vi "NumberDetector.vi"(1 "Array":dbl[](array[numeric])) -> (0 "f":string)   [LabVIEW 2020]
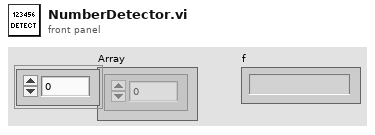
[diagram p1: front panel]
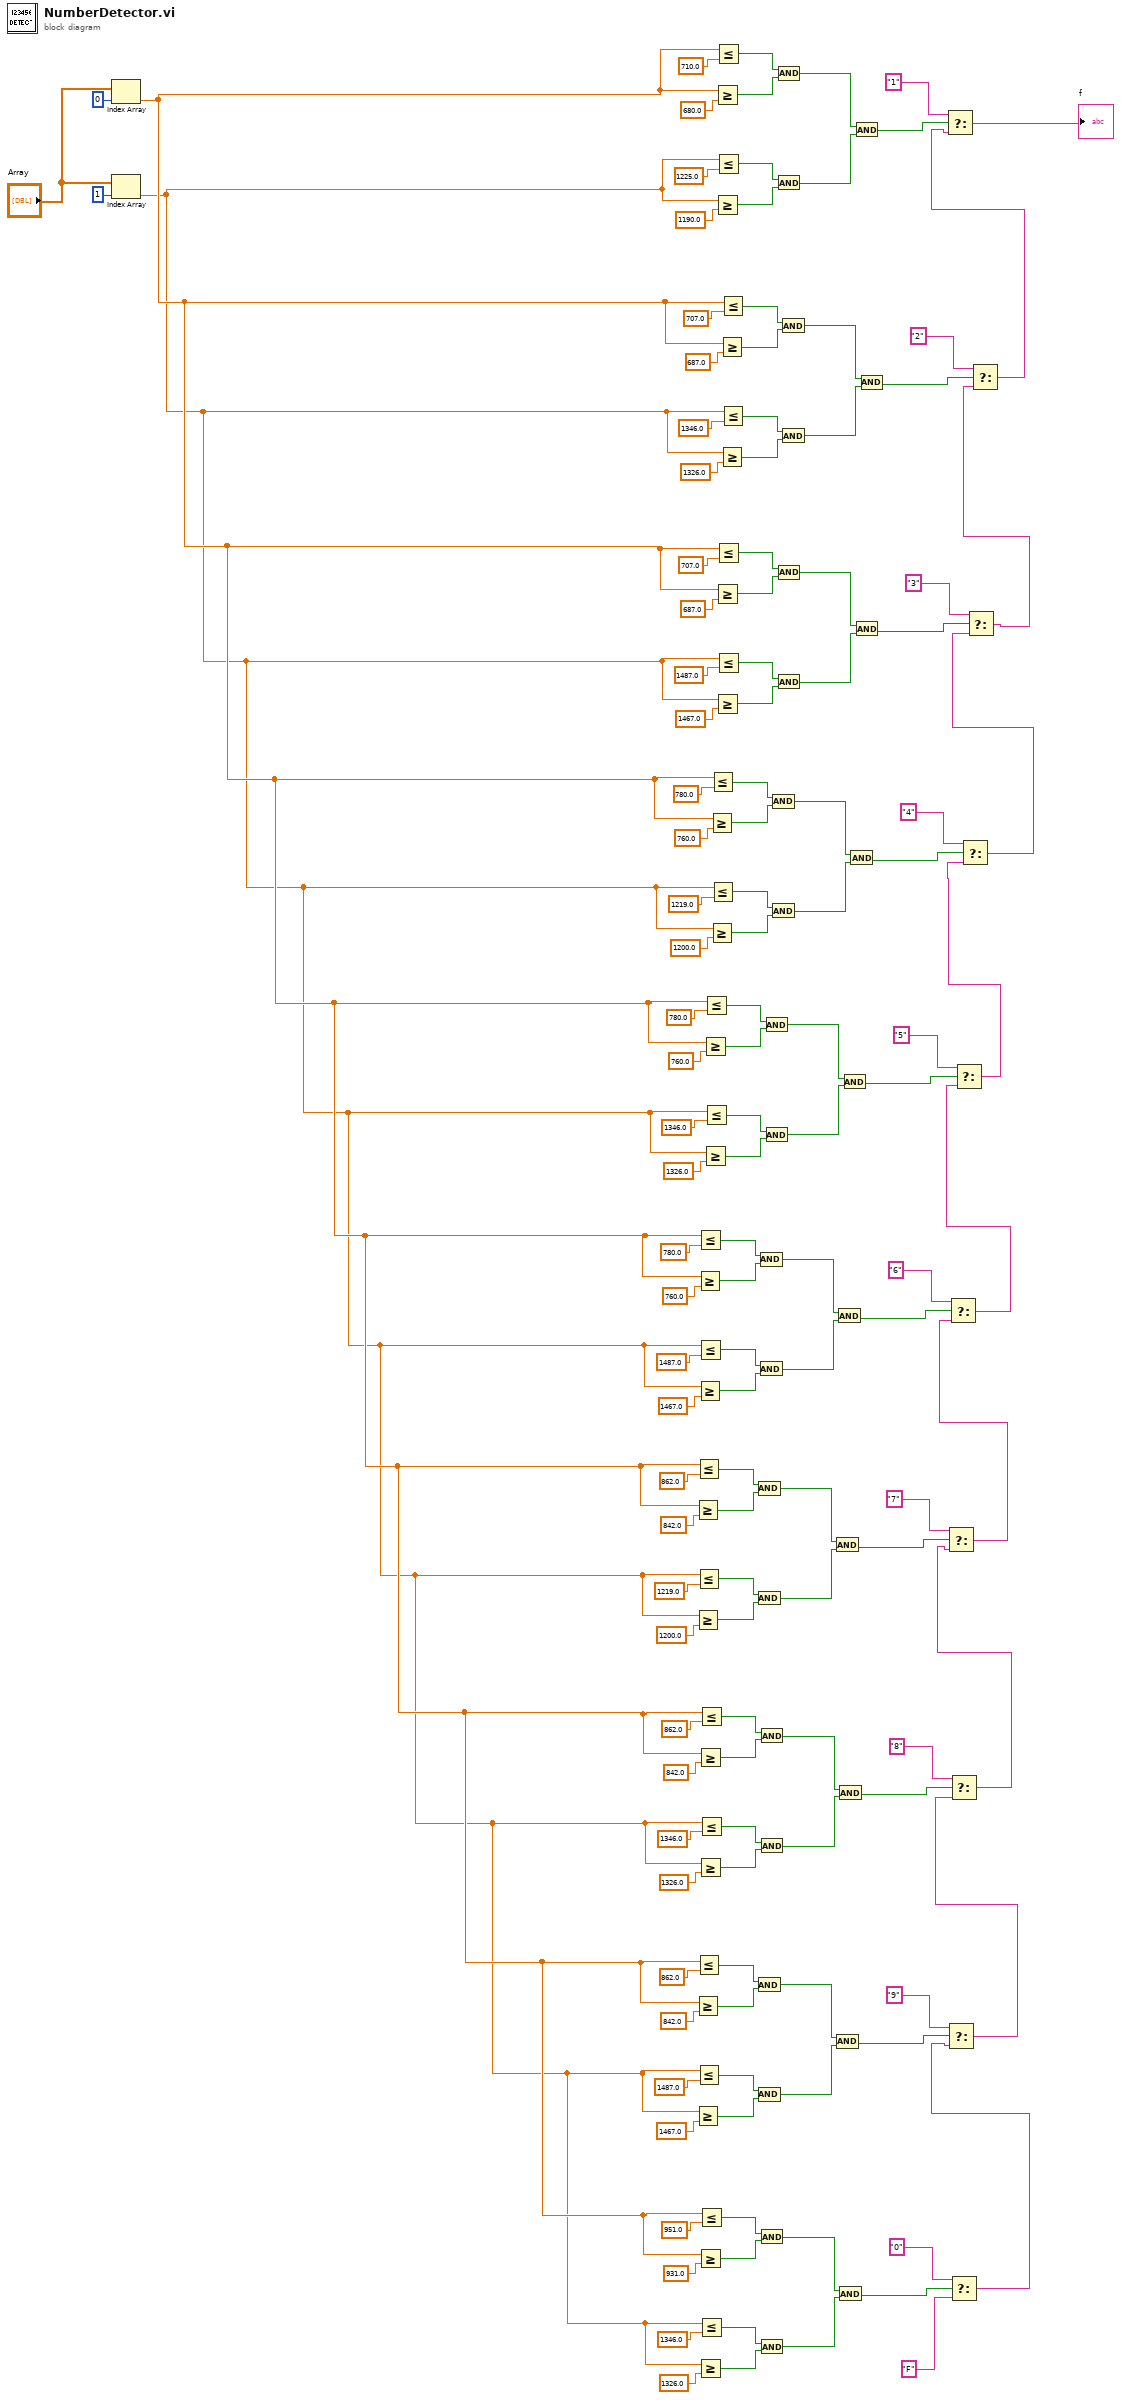
[diagram p0: block diagram]
diagram:
  n1 = Index Array(array="Array", index=0) -> (element=w4:dbl)
  n2 = Index Array(array="Array", index=1) -> (element=w3:dbl)
  n3 = Greater Or Equal?(x=w4, y=842.0) -> (x >= y?=w49:bool)
  n4 = Greater Or Equal?(x=w3, y=1200.0) -> (x >= y?=w50:bool)
  n5 = Greater Or Equal?(x=w4, y=842.0) -> (x >= y?=w23:bool)
  n6 = Greater Or Equal?(x=w3, y=1467.0) -> (x >= y?=w24:bool)
  n7 = Less Or Equal?(x=w4, y=862.0) -> (x <= y?=w48:bool)
  n8 = Less Or Equal?(x=w3, y=1219.0) -> (x <= y?=w51:bool)
  n9 = Less Or Equal?(x=w4, y=862.0) -> (x <= y?=w22:bool)
  n10 = Less Or Equal?(x=w3, y=1487.0) -> (x <= y?=w25:bool)
  n11 = Greater Or Equal?(x=w4, y=760.0) -> (x >= y?=w63:bool)
  n12 = Greater Or Equal?(x=w3, y=1467.0) -> (x >= y?=w62:bool)
  n13 = Less Or Equal?(x=w4, y=780.0) -> (x <= y?=w64:bool)
  n14 = Less Or Equal?(x=w3, y=1487.0) -> (x <= y?=w61:bool)
  n15 = Greater Or Equal?(x=w4, y=842.0) -> (x >= y?=w37:bool)
  n16 = Greater Or Equal?(x=w3, y=1326.0) -> (x >= y?=w36:bool)
  n17 = Greater Or Equal?(x=w4, y=931.0) -> (x >= y?=w11:bool)
  n18 = Greater Or Equal?(x=w3, y=1326.0) -> (x >= y?=w10:bool)
  n19 = Less Or Equal?(x=w4, y=862.0) -> (x <= y?=w38:bool)
  n20 = Less Or Equal?(x=w3, y=1346.0) -> (x <= y?=w35:bool)
  n21 = Less Or Equal?(x=w4, y=951.0) -> (x <= y?=w12:bool)
  n22 = Less Or Equal?(x=w3, y=1346.0) -> (x <= y?=w9:bool)
  n23 = Greater Or Equal?(x=w4, y=760.0) -> (x >= y?=w75:bool)
  n24 = Greater Or Equal?(x=w3, y=1326.0) -> (x >= y?=w76:bool)
  n25 = Less Or Equal?(x=w4, y=780.0) -> (x <= y?=w74:bool)
  n26 = Less Or Equal?(x=w3, y=1346.0) -> (x <= y?=w77:bool)
  n27 = Greater Or Equal?(x=w4, y=760.0) -> (x >= y?=w89:bool)
  n28 = Greater Or Equal?(x=w3, y=1200.0) -> (x >= y?=w88:bool)
  n29 = Less Or Equal?(x=w4, y=780.0) -> (x <= y?=w90:bool)
  n30 = Less Or Equal?(x=w3, y=1219.0) -> (x <= y?=w87:bool)
  n31 = Greater Or Equal?(x=w4, y=680.0) -> (x >= y?=w114:bool)
  n32 = Greater Or Equal?(x=w3, y=1190.0) -> (x >= y?=w115:bool)
  n33 = Greater Or Equal?(x=w4, y=687.0) -> (x >= y?=w101:bool)
  n34 = Greater Or Equal?(x=w3, y=1467.0) -> (x >= y?=w102:bool)
  n35 = Less Or Equal?(x=w4, y=710.0) -> (x <= y?=w113:bool)
  n36 = Less Or Equal?(x=w3, y=1225.0) -> (x <= y?=w116:bool)
  n37 = Less Or Equal?(x=w4, y=707.0) -> (x <= y?=w100:bool)
  n38 = Less Or Equal?(x=w3, y=1487.0) -> (x <= y?=w103:bool)
  n39 = Greater Or Equal?(x=w4, y=687.0) -> (x >= y?=w130:bool)
  n40 = Greater Or Equal?(x=w3, y=1326.0) -> (x >= y?=w129:bool)
  n41 = Less Or Equal?(x=w4, y=707.0) -> (x <= y?=w131:bool)
  n42 = Less Or Equal?(x=w3, y=1346.0) -> (x <= y?=w128:bool)
  n43 = And(x=w48, y=w49) -> (x .and. y?=w54:bool)
  n44 = And(x=w51, y=w50) -> (x .and. y?=w55:bool)
  n45 = And(x=w22, y=w23) -> (x .and. y?=w28:bool)
  n46 = And(x=w25, y=w24) -> (x .and. y?=w29:bool)
  n47 = And(x=w64, y=w63) -> (x .and. y?=w58:bool)
  n48 = And(x=w61, y=w62) -> (x .and. y?=w57:bool)
  n49 = And(x=w38, y=w37) -> (x .and. y?=w32:bool)
  n50 = And(x=w35, y=w36) -> (x .and. y?=w31:bool)
  n51 = And(x=w12, y=w11) -> (x .and. y?=w6:bool)
  n52 = And(x=w9, y=w10) -> (x .and. y?=w5:bool)
  n53 = And(x=w74, y=w75) -> (x .and. y?=w80:bool)
  n54 = And(x=w77, y=w76) -> (x .and. y?=w81:bool)
  n55 = And(x=w90, y=w89) -> (x .and. y?=w84:bool)
  n56 = And(x=w87, y=w88) -> (x .and. y?=w83:bool)
  n57 = And(x=w113, y=w114) -> (x .and. y?=w119:bool)
  n58 = And(x=w116, y=w115) -> (x .and. y?=w120:bool)
  n59 = And(x=w100, y=w101) -> (x .and. y?=w106:bool)
  n60 = And(x=w103, y=w102) -> (x .and. y?=w107:bool)
  n61 = And(x=w131, y=w130) -> (x .and. y?=w125:bool)
  n62 = And(x=w128, y=w129) -> (x .and. y?=w124:bool)
  n63 = And(x=w54, y=w55) -> (x .and. y?=w44:bool)
  n64 = And(x=w28, y=w29) -> (x .and. y?=w18:bool)
  n65 = And(x=w58, y=w57) -> (x .and. y?=w68:bool)
  n66 = And(x=w32, y=w31) -> (x .and. y?=w42:bool)
  n67 = And(x=w6, y=w5) -> (x .and. y?=w16:bool)
  n68 = And(x=w80, y=w81) -> (x .and. y?=w70:bool)
  n69 = And(x=w84, y=w83) -> (x .and. y?=w94:bool)
  n70 = And(x=w119, y=w120) -> (x .and. y?=w121:bool)
  n71 = And(x=w106, y=w107) -> (x .and. y?=w96:bool)
  n72 = And(x=w125, y=w124) -> (x .and. y?=w135:bool)
  n73 = Select(t="0", s=w16, f="F") -> (s? t:f=w1:string)
  n74 = Select(t="9", s=w18, f=w1) -> (s? t:f=w17:string)
  n75 = Select(t="8", s=w42, f=w17) -> (s? t:f=w30:string)
  n76 = Select(t="7", s=w44, f=w30) -> (s? t:f=w43:string)
  n77 = Select(t="6", s=w68, f=w43) -> (s? t:f=w56:string)
  n78 = Select(t="5", s=w70, f=w56) -> (s? t:f=w69:string)
  n79 = Select(t="4", s=w94, f=w69) -> (s? t:f=w82:string)
  n80 = Select(t="3", s=w96, f=w82) -> (s? t:f=w95:string)
  n81 = Select(t="2", s=w135, f=w95) -> (s? t:f=w136:string)
  n82 = Select(t="1", s=w121, f=w136) -> (s? t:f=→"f":string)
